vi "Fuel Refinement Fast.vi"() -> ()   [LabVIEW 2023]
uses:
  <vilib>/Utility/config.llb/NI_LVConfig.lvlib
  <vilib>/Utility/config.llb/Read Key (U32).vi
panel:
  in  "stop":bool
  in  "configuration file path":path
  in  "# Dissolution Chambers":u32=1 min=1
  out "H2SO4 Demand (mB/t)":ext format="%.2f"
  out "Yellow Cake Blocks/t":ext
  in  "Slots":u32=3 min=3 max=9 step=2
  in  "Chem. Dissolution Gas":u32 max=8
  out "UF6 Limiting":bool
  in  "Centrifuge Speed":u32 max=8
  out "UF6 (mB/t)":ext format="%.2f"
  out "Self Limiting":bool
  out "UO Limiting":bool
  out "HF Limiting":bool
  out "HF (mB/t)":ext format="%.2f"
  out "UO (mB/t)":ext format="%.2f"
  out "UF6 (mB/t)":ext format="%.2f"
  in  "Chem. Infuser Speed":u32 max=8
  out "Fluorite/s":ext
  out "Uranium Ingots/s":ext
  out "Yellow Cake/t":ext
  in  "Enrichment Speed":u32 max=8
  out "YK Limiting":bool
  out "Self Limiting":bool
  out "UO2 (mB/t)":ext format="%.2f"
  in  "Ox Speed":u32 max=8
  out "Coal Blocks/s":ext
  out "HF (mB/t)":u32
  out "H2SO4 Limiting":bool
  out "Self Limiting":bool
  out "H2SO4 (mB/t)":ext format="%.2f"
  in  "Chem. Dissolution Speed":u32 max=8
  out "Fluorite/t":ext
  out "Self Limiting":bool
  out "H2O Limiting":bool
  out "SO3 Limiting":bool
  out "SO3 (mB/t)":ext format="%.2f"
  out "H2O Vapor (mB/t)":ext format="%.2f"
  out "Sulfur Dust/t":ext
  out "H2SO4 (mB/t)":ext format="%.2f"
  in  "Chem. Infuser Speed":u32 max=8
  out "H2O Vapor (mB/t)":u32
  in  "Rotary Cond. Speed":u32 max=8
  out "SO3 (mB/t)":ext format="%.2f"
  out "Self Limiting":bool
  out "SO2 Limiting":bool
  out "O Limiting":bool
  out "O (mB/t)":ext format="%.2f"
  out "SO2 (mB/t)":ext format="%.2f"
  in  "Chem. Infuser Speed":u32 max=8
  out "H (mB/t)":u32
  out "O (mB/t)":u32
  in  "E.S. Speed":u32 max=8
  out "Dust Limiting":bool
  out "Self Limiting":bool
  out "SO2 (mB/t)":ext format="%.2f"
  in  "Ox Speed":u32 max=8
  out "H (mB/t)":u32
  out "O (mB/t)":u32
  out "Self Limiting":bool
  out "PRC O Limiting":bool
  out "PRC H2O Limiting":bool
  in  "P.R.C. Speed":u32 max=8
  in  "E.S. Speed":u32 max=8
  out "Coal Blocks/t":ext
  out "Self Limiting":bool
  out "Fissile Fuel (mB/t)":ext
  out "Uranium Ingots/t":ext
  # "Input Requirements"
  # "Sulfur Elec. Separator"
  # "Sulfur Elec. Separator"
  # "Water Vapor"
  # "Input Requirements"
  # "Sulfur Production"
  # "Sulfur Dioxide"
  # "Sulfur Trixoide"
  # "Sulfuric Acid"
  # "Yellow Cake Production"
  # "Uranium Oxide"
  # "Uranium Hexafluoride"
  # "Hydrofluoric Acid"
  # "Fissile Fuel"
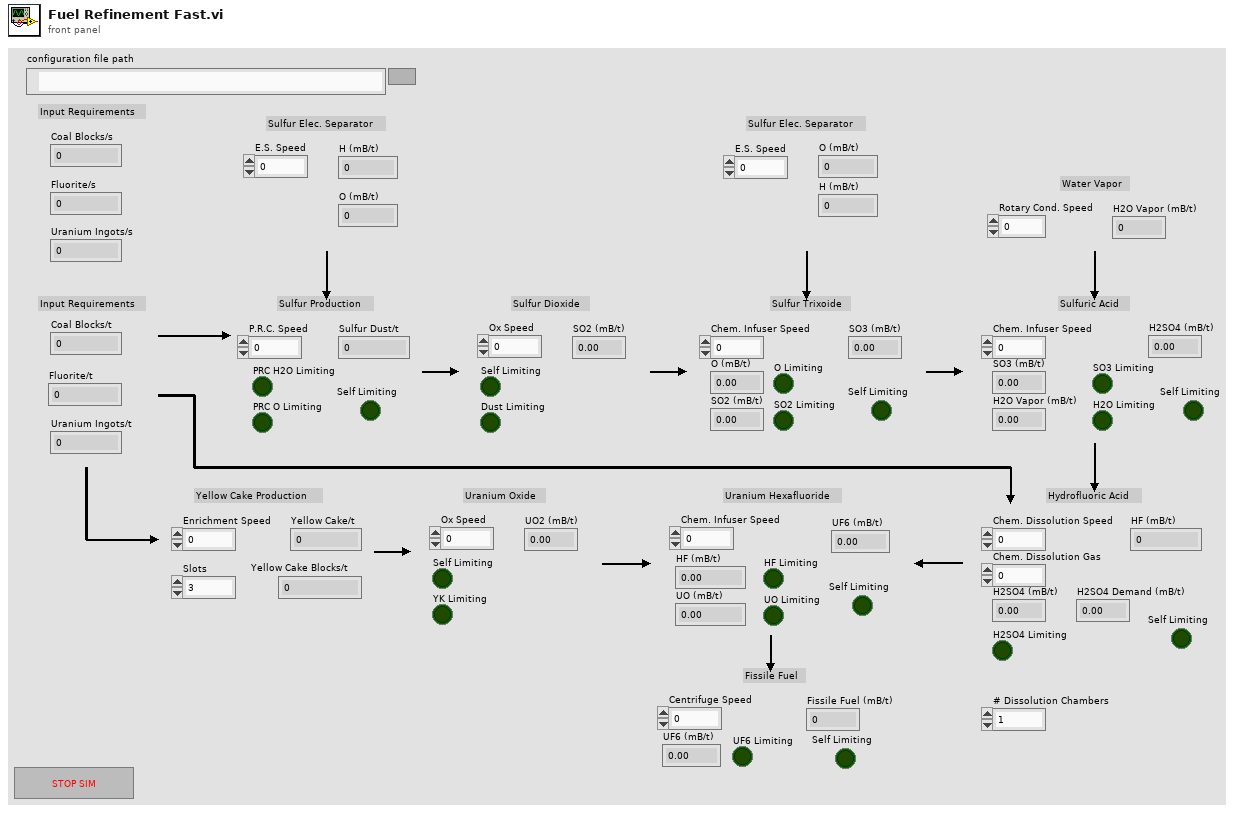
[diagram p1: front panel]
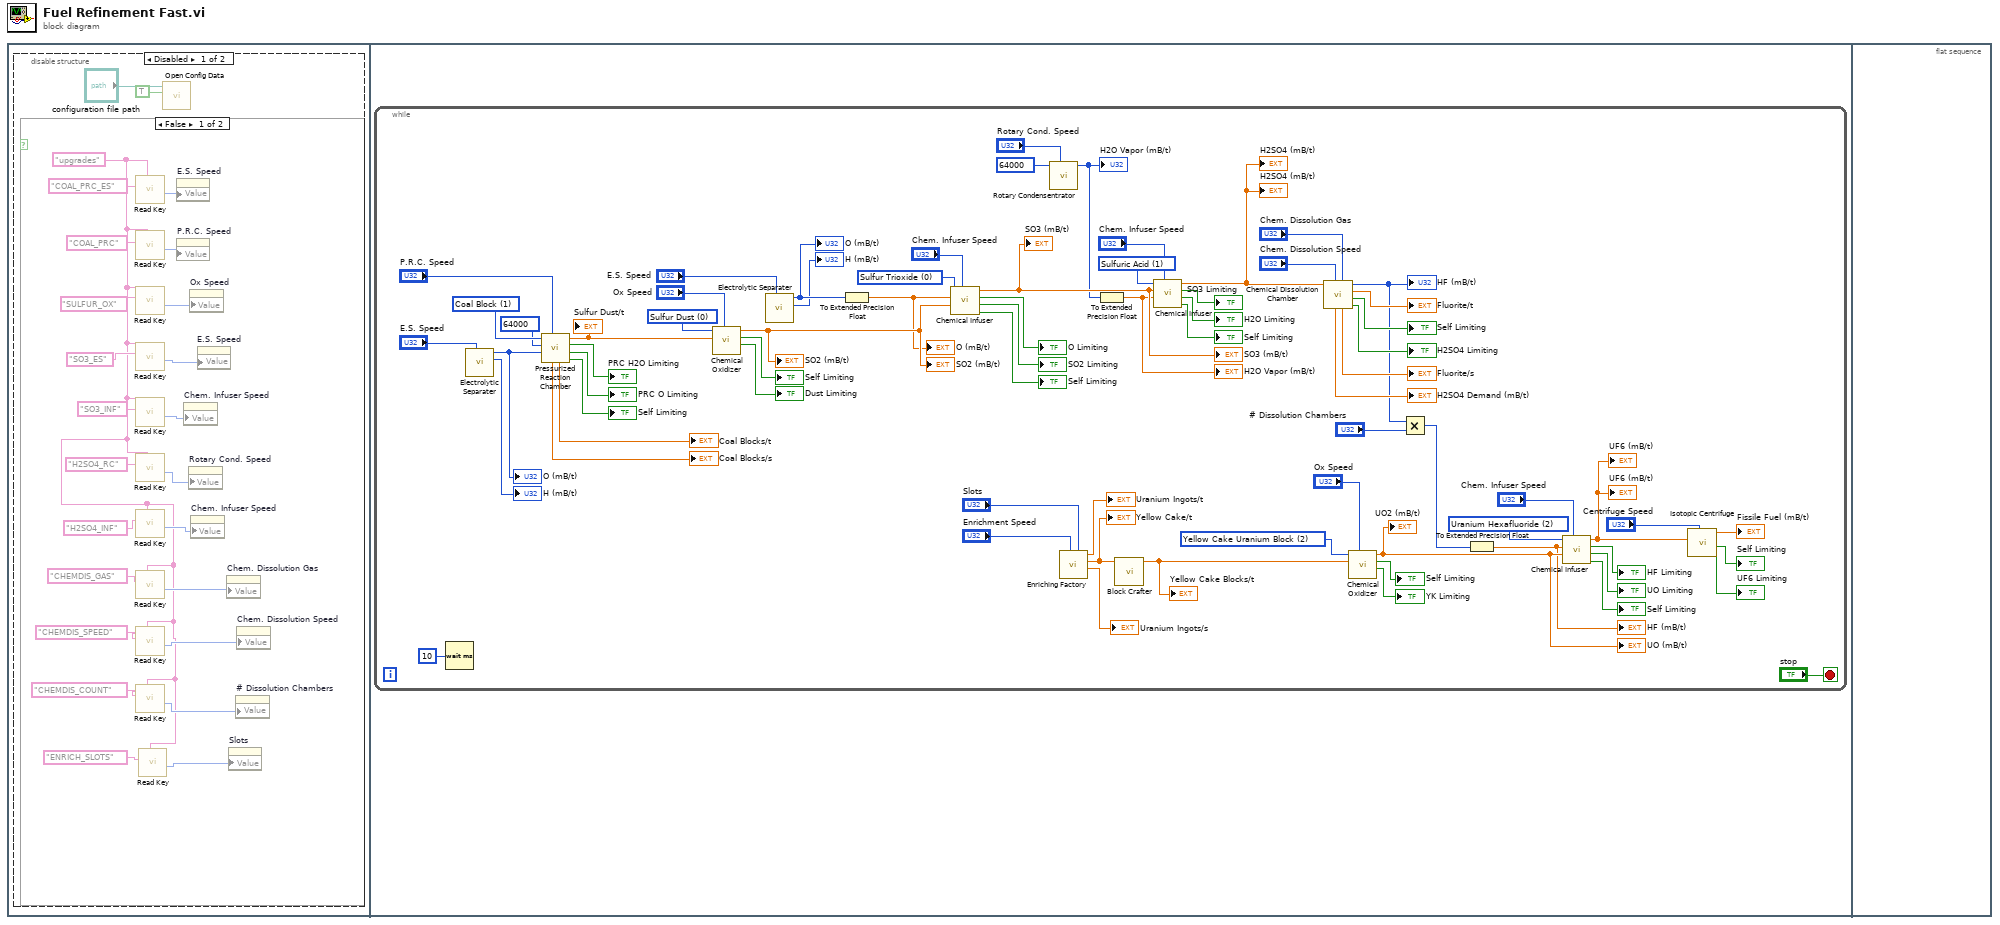
[diagram p0: block diagram]
diagram:
  n1 = flat-sequence {
    frame #0 {
      n2 = disable-structure shown="Disabled" {
        frame Disabled {
          n3 = case shown="False" {
            selector: _ -> [_ _]
            frame False {
              w5 = "upgrades" ("section")
              n4 = call-poly <vilib>:"Read Key.vi"("section"=w5, "key"="COAL_PRC_ES") -> ("value"=w24:u32)  [unwired: 6 in, 3 out]
              n5 = call-poly <vilib>:"Read Key.vi"("section"=w5, "key"="COAL_PRC") -> ("value"=w22:u32)  [unwired: 6 in, 3 out]
              n6 = call-poly <vilib>:"Read Key.vi"("section"=w5, "key"="SULFUR_OX") -> ("value"=w18:u32)  [unwired: 6 in, 3 out]
              n7 = call-poly <vilib>:"Read Key.vi"("section"=w5, "key"="SO3_ES") -> ("value"=w19:u32)  [unwired: 6 in, 3 out]
              n8 = call-poly <vilib>:"Read Key.vi"("section"=w5, "key"="SO3_INF") -> ("value"=w16:u32)  [unwired: 6 in, 3 out]
              n9 = call-poly <vilib>:"Read Key.vi"("section"=w5, "key"="H2SO4_RC") -> ("value"=w15:u32)  [unwired: 6 in, 3 out]
              n10 = call-poly <vilib>:"Read Key.vi"("section"=w5, "key"="H2SO4_INF") -> ("value"=w12:u32)  [unwired: 6 in, 3 out]
              n11 = call-poly <vilib>:"Read Key.vi"("section"=w5, "key"="CHEMDIS_GAS") -> ("value"=w10:u32)  [unwired: 6 in, 3 out]
              n12 = call-poly <vilib>:"Read Key.vi"("section"=w5, "key"="CHEMDIS_SPEED") -> ("value"=w8:u32)  [unwired: 6 in, 3 out]
              n13 = call-poly <vilib>:"Read Key.vi"("section"=w5, "key"="CHEMDIS_COUNT") -> ("value"=w6:u32)  [unwired: 6 in, 3 out]
              n14 = call-poly <vilib>:"Read Key.vi"("section"=w5, "key"="ENRICH_SLOTS") -> ("value"=w3:u32)  [unwired: 6 in, 3 out]
              n15 = property on="E.S. Speed" class="DigNum (strict)"("Value"=w24) -> ()  [unwired: 2 in, 2 out]
              n16 = property on="P.R.C. Speed" class="DigNum (strict)"("Value"=w22) -> ()  [unwired: 2 in, 2 out]
              n17 = property on="Chem. Infuser Speed" class="DigNum (strict)"("Value"=w16) -> ()  [unwired: 2 in, 2 out]
              n18 = property on="Rotary Cond. Speed" class="DigNum (strict)"("Value"=w15) -> ()  [unwired: 2 in, 2 out]
              n19 = property on="Ox Speed" class="DigNum (strict)"("Value"=w18) -> ()  [unwired: 2 in, 2 out]
              n20 = property on="Chem. Infuser Speed" class="DigNum (strict)"("Value"=w12) -> ()  [unwired: 2 in, 2 out]
              n21 = property on="E.S. Speed" class="DigNum (strict)"("Value"=w19) -> ()  [unwired: 2 in, 2 out]
              n22 = property on="Chem. Dissolution Gas" class="DigNum (strict)"("Value"=w10) -> ()  [unwired: 2 in, 2 out]
              n23 = property on="Slots" class="DigNum (strict)"("Value"=w3) -> ()  [unwired: 2 in, 2 out]
              n24 = property on="# Dissolution Chambers" class="DigNum (strict)"("Value"=w6) -> ()  [unwired: 2 in, 2 out]
              n25 = property on="Chem. Dissolution Speed" class="DigNum (strict)"("Value"=w8) -> ()  [unwired: 2 in, 2 out]
            }
            frame True {
            }
          }
          n26 = call <vilib>:"Open Config Data.vi"("create file if necessary (T)"=TRUE, "configuration file path"="configuration file path") -> ()  [unwired: 7 in, 3 out]
        }
        frame Enabled {
        }
      }
    }
    frame #1 {
      n27 = while {
        stop <- "stop" stop-if-true
        w86 = u16 0 items=["Sulfur Trioxide", "Sulfuric Acid", "Uranium Hexafluoride"] ("Recipe")
        w89 = u16 0 items=["Sulfur Dust", "Yellow Cake Uranium", "Yellow Cake Uranium Block"] ("Input")
        w92 = u16 1 items=["Sulfur Trioxide", "Sulfuric Acid", "Uranium Hexafluoride"] ("Recipe")
        w93 = u16 2 items=["Sulfur Trioxide", "Sulfuric Acid", "Uranium Hexafluoride"] ("Recipe")
        w95 = u16 1 items=["Coal", "Coal Block"] ("Input")
        w96 = u16 2 items=["Sulfur Dust", "Yellow Cake Uranium", "Yellow Cake Uranium Block"] ("Input")
        n28 = Wait (ms)(milliseconds to wait=u32 10) -> ()  [unwired: 1 out]
        n29 = call "Electrolytic Separater.vi"("Speed Upgrades"="E.S. Speed") -> ("Hydrogen (mB/t)"=→"H (mB/t)":u32, "Oxygen (mB/t)"=w88:u32)  [unwired: 6 in]
        "O (mB/t)" <- w88
        n30 = call "Pressurized Reaction Chamber.vi"("Speed Upgrades"="P.R.C. Speed", "In Gas (mB/t)"=w88, "Water (mB/t)"=u32 64000, "Input"=w95) -> ("Limiting"=→"Self Limiting":bool, "B Limiting"=→"PRC O Limiting":bool, "A Limiting"=→"PRC H2O Limiting":bool, "Produced Items/t"=w32:ext, "Required Items/t"=→"Coal Blocks/t":ext, "Required Items/s"=→"Coal Blocks/s":ext)  [unwired: 1 in, 1 out]
        "Sulfur Dust/t" <- w32
        n31 = call "Chemical Oxidizer.vi"("Speed Upgrades"="Ox Speed", "Items/t In"=w32, "Input"=w89) -> ("Input Limiting"=→"Dust Limiting":bool, "Limiting"=→"Self Limiting":bool, "Output Gas (mB/t)"=w39:ext)  [unwired: 4 in, 2 out]
        "SO2 (mB/t)" <- w39
        "SO2 (mB/t)" <- w39
        n32 = call "Electrolytic Separater.vi"("Speed Upgrades"="E.S. Speed") -> ("Hydrogen (mB/t)"=→"H (mB/t)":u32, "Oxygen (mB/t)"=w85:u32)  [unwired: 6 in]
        "O (mB/t)" <- w85
        n33 = To Extended Precision Float(1:w85) -> (0:w38:ext)
        "O (mB/t)" <- w38
        n34 = call "Chemical Infuser.vi"("Speed Upgrades"="Chem. Infuser Speed", "Gas B (mB/t)"=w39, "Gas A (mB/t)"=w38, "Recipe"=w86) -> ("Limiting"=→"Self Limiting":bool, "B Limiting"=→"SO2 Limiting":bool, "A Limiting"=→"O Limiting":bool, "Output Gas (mB/t)"=w62:ext)  [unwired: 4 in]
        "SO3 (mB/t)" <- w62
        "SO3 (mB/t)" <- w62
        n35 = call "Rotary Condensentrator.vi"("Speed Upgrades"="Rotary Cond. Speed", "Liquid (mB/t)"=u32 64000) -> ("Gas (mB/t)"=w61:u32)  [unwired: 8 in, 1 out]
        "H2O Vapor (mB/t)" <- w61
        n36 = call "Enriching Factory.vi"("Slots"="Slots", "Speed Upgrades"="Enrichment Speed") -> ("Uranium Ingots/s"=→"Uranium Ingots/s":ext, "Yellow Cake/t"=w34:ext, "Uranium Ingots/t"=→"Uranium Ingots/t":ext)  [unwired: 6 in, 1 out]
        "Yellow Cake/t" <- w34
        n37 = To Extended Precision Float(1:w61) -> (0:w37:ext)
        "H2O Vapor (mB/t)" <- w37
        n38 = call "Block Crafter.vi"("In Items/t"=w34) -> ("Out Items/t"=w33:ext)  [unwired: 8 in]
        "Yellow Cake Blocks/t" <- w33
        n39 = call "Chemical Infuser.vi"("Speed Upgrades"="Chem. Infuser Speed", "Gas B (mB/t)"=w37, "Gas A (mB/t)"=w62, "Recipe"=w92) -> ("Limiting"=→"Self Limiting":bool, "B Limiting"=→"H2O Limiting":bool, "A Limiting"=→"SO3 Limiting":bool, "Output Gas (mB/t)"=w36:ext)  [unwired: 4 in]
        "H2SO4 (mB/t)" <- w36
        "H2SO4 (mB/t)" <- w36
        n40 = call "Chemical Dissolution Chamber.vi"("Gas Upgrades"="Chem. Dissolution Gas", "Speed Upgrades"="Chem. Dissolution Speed", "Sulfuric Acid (mB/t)"=w36) -> ("Input Limiting"=→"H2SO4 Limiting":bool, "Limiting"=→"Self Limiting":bool, "Required Items/t"=→"Fluorite/t":ext, "Hydrofluoric Acid (mB/t)"=w30:u32, "Required Items/s"=→"Fluorite/s":ext, "Gas Required (mB/t)"=→"H2SO4 Demand (mB/t)":ext)  [unwired: 3 in]
        "HF (mB/t)" <- w30
        n41 = call "Chemical Oxidizer.vi"("Speed Upgrades"="Ox Speed", "Items/t In"=w33, "Input"=w96) -> ("Input Limiting"=→"YK Limiting":bool, "Limiting"=→"Self Limiting":bool, "Output Gas (mB/t)"=w41:ext)  [unwired: 4 in, 2 out]
        "UO2 (mB/t)" <- w41
        "UO (mB/t)" <- w41
        n42 = Multiply(x=w30, y="# Dissolution Chambers") -> (x*y=w28:u32)
        n43 = To Extended Precision Float(1:w28) -> (0:w40:ext)
        "HF (mB/t)" <- w40
        n44 = call "Chemical Infuser.vi"("Speed Upgrades"="Chem. Infuser Speed", "Gas B (mB/t)"=w41, "Gas A (mB/t)"=w40, "Recipe"=w93) -> ("Limiting"=→"Self Limiting":bool, "B Limiting"=→"UO Limiting":bool, "A Limiting"=→"HF Limiting":bool, "Output Gas (mB/t)"=w45:ext)  [unwired: 4 in]
        "UF6 (mB/t)" <- w45
        "UF6 (mB/t)" <- w45
        n45 = call "Isotopic Centrifuge.vi"("Speed Upgrades"="Centrifuge Speed", "Uranium Hexaflouride (mB/t)"=w45) -> ("Input Limiting"=→"UF6 Limiting":bool, "Limiting"=→"Self Limiting":bool, "Fissile Fuel (mB/t)"=→"Fissile Fuel (mB/t)":ext)  [unwired: 4 in]
      }
    }
    frame #2 {
    }
  }
